vi "DSF.Engine.Interface.New.vi"(7 "fifo depths (10)":u32, 8 "error in (no error)":errorcluster, 11 "Interface type":refnum<class "DSF.Engine.Interface.lvclass">) -> (0 "error out":errorcluster, 3 "Interface":refnum<class "DSF.Engine.Interface.lvclass">)   [LabVIEW 2016, in "DSF.Engine.lvlib" / "DSF.Engine.Interface.lvclass"]
uses:
  DSF.Engine.Interface.lvclass
  DSF.Engine.Interface.lvclass/DSF.Engine.Interface.ctl
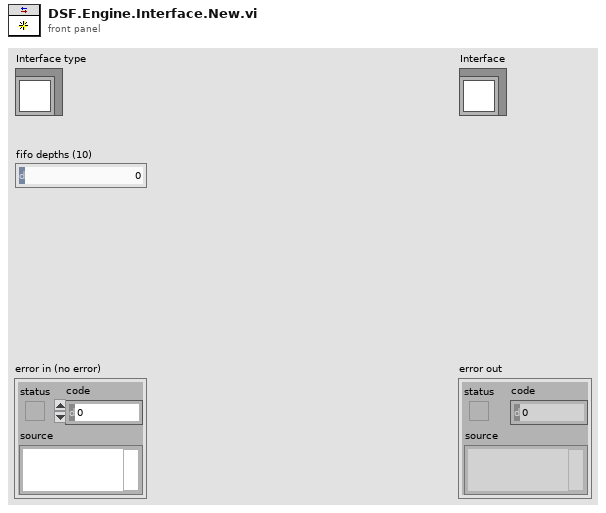
[diagram p1: front panel]
types:
  T1 = typedef "DSF.Engine.lvlib/DSF.Engine.Interface.lvclass/DSF.Engine.Interface.RT FIFO Ref.ctl" = refnum<k33>
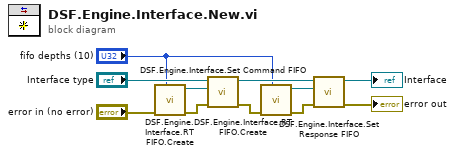
[diagram p0: block diagram]
diagram:
  n1 = call "DSF.Engine.Interface.RT FIFO.Create.vi"("size (10)"="fifo depths (10)", "error in (no error)"="error in (no error)") -> ("error out"=w10:errorcluster, "RT FIFO"=w5:T1)  [unwired: 8 in]
  n2 = call "DSF.Engine.Interface.Set Command FIFO.vi"("error in (no error)"=w10, "Command FIFO"=w5, "Interface in"="Interface type") -> ("error out"=w9:errorcluster, "Interface out"=w2:refnum<class "DSF.Engine.Interface.lvclass">)  [unwired: 7 in]
  n3 = call "DSF.Engine.Interface.RT FIFO.Create.vi"("size (10)"="fifo depths (10)", "error in (no error)"=w9) -> ("error out"=w8:errorcluster, "RT FIFO"=w4:T1)  [unwired: 8 in]
  n4 = call "DSF.Engine.Interface.Set Response FIFO.vi"("error in (no error)"=w8, "Response FIFO"=w4, "Interface in"=w2) -> ("error out"=→"error out":errorcluster, "Interface out"=→"Interface":refnum<class "DSF.Engine.Interface.lvclass">)  [unwired: 7 in]
